vi "FireMessageEvent.vi"(0 "object in":refnum<class "Application.lvclass">, 1 "Message":string, 3 "Message Data":variant, 5 "error in (no error)":errorcluster) -> (14 "object out":refnum<class "Application.lvclass">, 19 "error out":errorcluster)   [LabVIEW 2021, in "Application.lvclass"]
uses:
  Application.lvclass
  Application.lvclass/Application.ctl
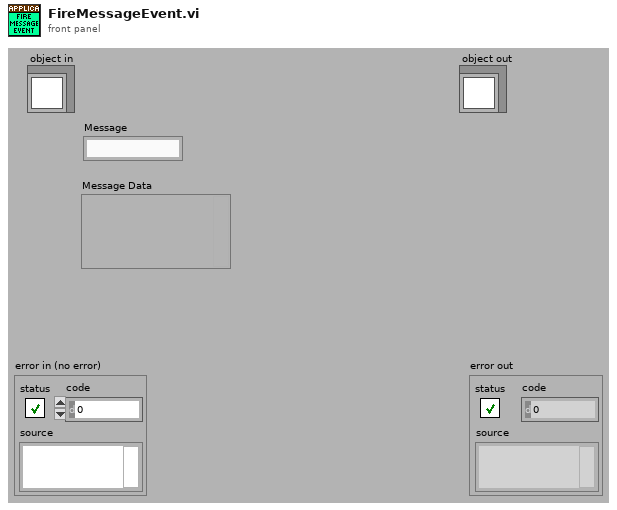
[diagram p1: front panel]
types:
  T1 = cluster{"Message":string, "Message Data":variant}
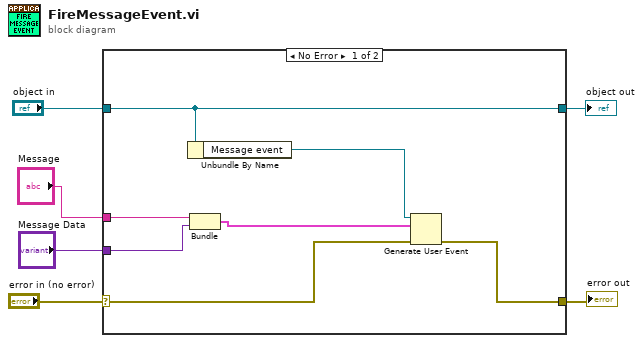
[diagram p0: block diagram]
diagram:
  n1 = case shown="No Error" "error in (no error)" {
    selector: "error in (no error)" -> [w11 w15]
    tunnel: [w10 w15] -> w5
    tunnel: [w13 w14] -> w3
    tunnel: "object in" -> [w13 w14]
    tunnel: "Message" -> [w9 _]
    tunnel: "Message Data" -> [w8 _]
    frame No Error {
      n2 = Unbundle By Name(w13) -> ("Message event"=w12:refnum<user-event>)
      n3 = Bundle("Message"=w9, "Message Data"=w8) -> (w7:T1)  [unwired: 1 in]
      n4 = Generate User Event(user event=w12, event data cluster=w7, error in=w11) -> (error out=w10:errorcluster)  [unwired: 1 in, 1 out]
    }
    frame Error {
    }
  }
  "error out" <- w5
  "object out" <- w3
